vi "DSF.Engine.Execution.Transfer.Set Buffer.vi"(8 "error in (no error)":errorcluster, 10 "Buffer":refnum<class "DSF.Engine.Memory.Buffer.lvclass">, 11 "Transfer in":refnum<class "DSF.Engine.Execution.Transfer.lvclass">) -> (0 "error out":errorcluster, 3 "Transfer out":refnum<class "DSF.Engine.Execution.Transfer.lvclass">)   [LabVIEW 2016, in "DSF.Engine.lvlib" / "DSF.Engine.Execution.Transfer.lvclass"]
uses:
  DSF.Engine.Execution.Transfer.lvclass
  Buffer/DSF.Engine.Memory.Buffer.lvclass
  DSF.Engine.Execution.Transfer.lvclass/DSF.Engine.Execution.Transfer.ctl
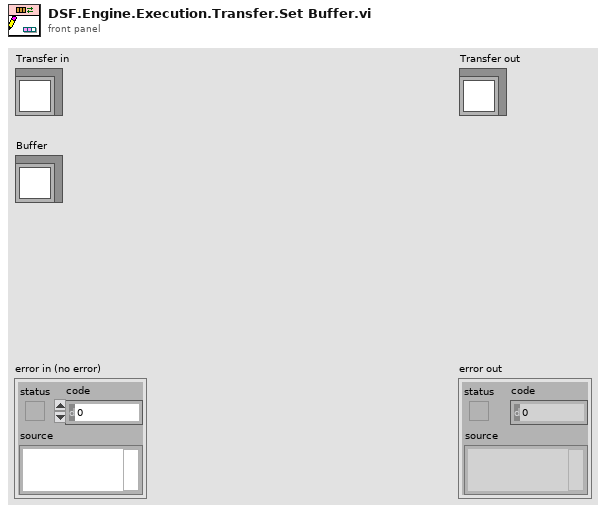
[diagram p1: front panel]
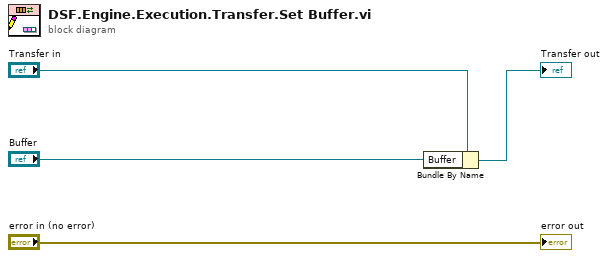
[diagram p0: block diagram]
diagram:
  n1 = Bundle By Name(cluster="Transfer in", "Buffer"="Buffer") -> (→"Transfer out":refnum<class "DSF.Engine.Execution.Transfer.lvclass">)
  "error out" <- "error in (no error)"
